vi "AlliGator Create Max & Sum Images.vi"(5 "Prefix":string, 6 "Image Characteristics":T2 {"Calibration"."Y Step" format="%.2f"; "Calibration"."X Step" format="%.2f"; "Image Type" items=["Grayscale (U8)", "Grayscale (I16)", "Grayscale (SGL)", "Complex (CSG)", "RGB (U32)", "HSL (U32)", "RGB (U64)", "Grayscale (U16)"]}, 7 "Image Type":bool, 8 "Error In":errorcluster, 9 "Image Min":T1, 10 "Image Max":T1, 11 "Image Sum":T1) -> (0 "Error Out":errorcluster, 1 "Image Min":T1, 2 "Image Max":T1, 3 "Image Sum":T1)   [LabVIEW 2021, in "AlliGator Files.lvlib"]
doc: "Creates image structures for Sum, Min and Max images"
uses:
  AlliGator Files.lvlib
  <vilib>/vision/Image Controls.llb/IMAQ Image.ctl
  Image/Image Characteristics.ctl
  Image/Image.lvlib
panel:
  # "see the AlliGator License on the block diagram (Ctrl+E or Window:Show Block Diagram)"
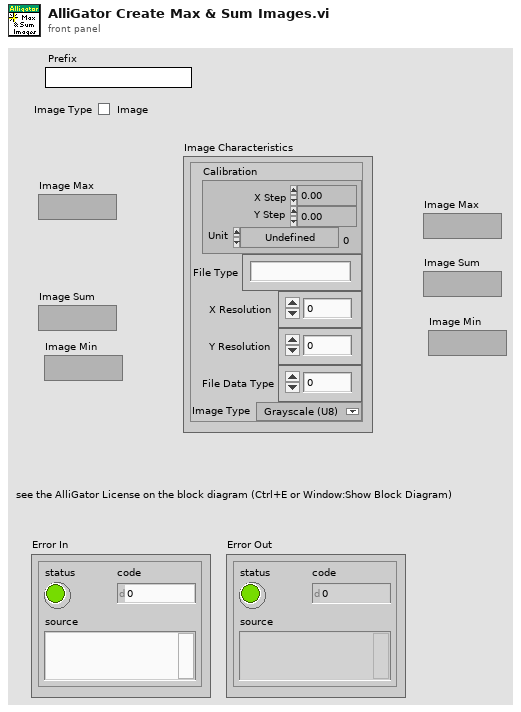
[diagram p1: front panel]
types:
  T1 = typedef "IMAQ Image.ctl" = refnum<image>
  T2 = typedef "Image.lvlib/Image Characteristics.ctl" = cluster{"Calibration":T3, "File Type":string, "X Resolution":i32, "Y Resolution":i32, "File Data Type":i32, "Image Type":T5}
  T3 = typedef "Simple Grid Descriptor" = cluster{"X Step":sgl, "Y Step":sgl, "Unit":T4}
  T4 = typedef "Image Unit" = enum32{"Undefined", "Angström", "Micrometer", "Millimeter", "Centimeter", "Meter", "Kilometer", "Microinch", "Inch", "Feet", "Nautical miles", "Standard miles", "Steps"}
  T5 = typedef "Image Type" = u32
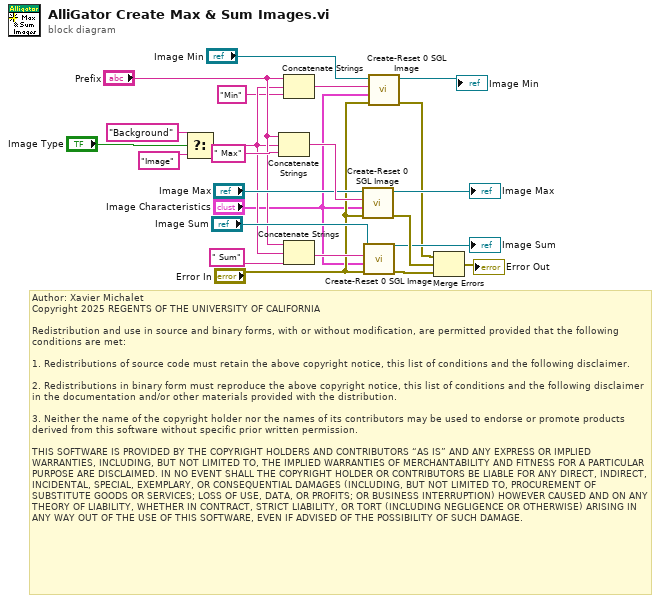
[diagram p0: block diagram]
diagram:
  # "Author: Xavier Michalet\nCopyright 2025 REGENTS OF THE UNIVERSITY OF CALIFORNIA\n\nRedistribution and use in source and binary forms, with or without modification, are permitted provided that the following conditions are met:\n\n1. Redistributions of source code must retain the above copyright notice, this list of conditions and the following disclaimer.\n\n2. Redistributions in binary form must reproduce the above copyright notice, this list of conditions and the following disclaimer in the documentation and/or other materials provided with the distribution.\n\n3. Neither the name of the copyright holder nor the names of its contributors may be used to endorse or promote products derived from this software without specific prior written permission.\n\nTHIS SOFTWARE IS PROVIDED BY THE COPYRIGHT HOLDERS AND CONTRIBUTORS “AS IS” AND ANY EXPRESS OR IMPLIED WARRANTIES, INCLUDING, BUT NOT LIMITED TO, THE IMPLIED WARRANTIES OF MERCHANTABILITY AND FITNESS FOR A PARTICULAR PURPOSE ARE DISCLAIMED. IN NO EVENT SHALL THE COPYRIGHT HOLDER OR CONTRIBUTORS BE LIABLE FOR ANY DIRECT, INDIRECT, INCIDENTAL, SPECIAL, EXEMPLARY, OR CONSEQUENTIAL DAMAGES (INCLUDING, BUT NOT LIMITED TO, PROCUREMENT OF SUBSTITUTE GOODS OR SERVICES; LOSS OF USE, DATA, OR PROFITS; OR BUSINESS INTERRUPTION) HOWEVER CAUSED AND ON ANY THEORY OF LIABILITY, WHETHER IN CONTRACT, STRICT LIABILITY, OR TORT (INCLUDING NEGLIGENCE OR OTHERWISE) ARISING IN ANY WAY OUT OF THE USE OF THIS SOFTWARE, EVEN IF ADVISED OF THE POSSIBILITY OF SUCH DAMAGE."
  n1 = Select(t="Background" ("x"), s="Image Type", f="Image") -> (s? t:f=w8:string)
  n2 = Concatenate Strings("Prefix", w8, " Max" ("Image Name")) -> (w21:string)
  n3 = Concatenate Strings("Prefix", w8, "Min" ("string")) -> (w6:string)
  n4 = Concatenate Strings("Prefix", w8, " Sum" ("Image Name")) -> (w22:string)
  n5 = call "Create-Reset 0 SGL Image.vi"("Error In"="Error In", "Image Characteristics"="Image Characteristics", "Image Name"=w21, "Image"="Image Max") -> ("Error Out"=w19:errorcluster, "New Image"=→"Image Max":T1)  [unwired: 6 in]
  n6 = call "Create-Reset 0 SGL Image.vi"("Error In"="Error In", "Image Characteristics"="Image Characteristics", "Image Name"=w22, "Image"="Image Sum") -> ("Error Out"=w18:errorcluster, "New Image"=→"Image Sum":T1)  [unwired: 6 in]
  n7 = call "Create-Reset 0 SGL Image.vi"("Error In"="Error In", "Image Characteristics"="Image Characteristics", "Image Name"=w6, "Image"="Image Min") -> ("Error Out"=w4:errorcluster, "New Image"=→"Image Min":T1)  [unwired: 6 in]
  n8 = Merge Errors(w4, w19, w18) -> (→"Error Out":errorcluster)
